vi "Init.vi"(8 "error in (no error)":errorcluster) -> (0 "error out":errorcluster, 3 "Controller out":refnum<class "Controller.lvclass">)   [LabVIEW 2020, in "Controller.lvlib" / "Controller.lvclass"]
uses:
  Controller.lvclass
  RPC/TypeDefs/Response.ctl
  Controller.lvclass/Controller.ctl
  RPC.lvlib
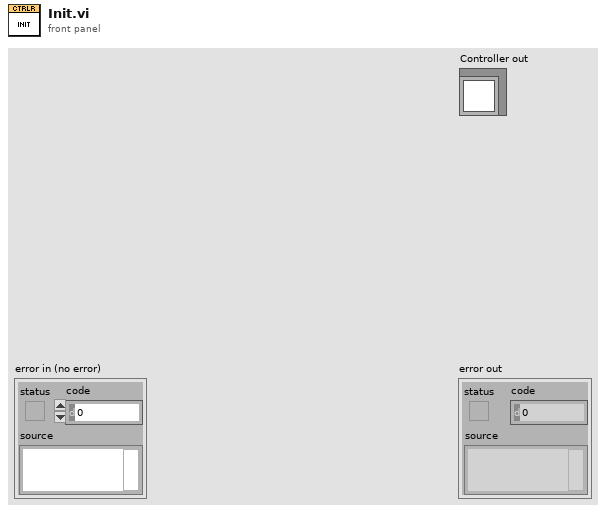
[diagram p1: front panel]
types:
  T1 = typedef "RPC.lvlib/Response.ctl" = cluster{"ID":string, "Response":variant}
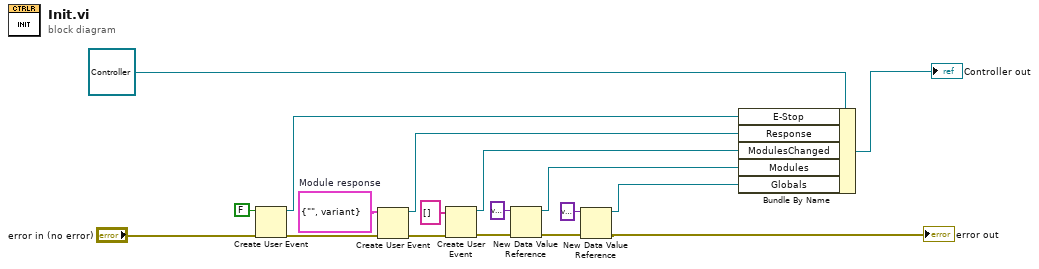
[diagram p0: block diagram]
diagram:
  w3 = T1 {"ID"="", "Response"=variant}  # Module response
  n1 = Create User Event(user event datatype=FALSE ("Stop Event"), error in="error in (no error)") -> (user event=w6:refnum<user-event>, error out=w4:errorcluster)
  n2 = Create User Event(user event datatype=w3, error in=w4) -> (user event=w2:refnum<user-event>, error out=w5:errorcluster)
  n3 = Create User Event(user event datatype=string[] [] ("Names"), error in=w5) -> (user event=w10:refnum<user-event>, error out=w12:errorcluster)
  n4 = New Data Value Reference(data value=variant, error in=w12) -> (data value reference=w9:refnum<data-value>, error out=w13:errorcluster)
  n5 = New Data Value Reference(data value=variant, error in=w13) -> (data value reference=w8:refnum<data-value>, error out=→"error out":errorcluster)
  n6 = Bundle By Name(cluster=refnum<class "Controller.lvclass"> refnum ("Controller in"), "E-Stop"=w6, "Response"=w2, "ModulesChanged"=w10, "Modules"=w9, "Globals"=w8) -> (→"Controller out":refnum<class "Controller.lvclass">)
